vi "Point Style Read.vi"(4 "error in (no error)":errorcluster, 6 "Container State":T3, 7 "Display State In":T1) -> (0 "error out":errorcluster, 2 "Value":u8, 3 "Display State Out":T1)   [LabVIEW 2020, in "XY Plot Matrix.xctl"]
uses:
  <vilib>/Math Plots/2D Math Plots/XY Plot Matrix/XY Plot Matrix XCtrl/XY Plot Matrix.xctl
  <vilib>/_xctls/Container State.ctl
  <vilib>/Math Plots/2D Math Plots/XY Plot Matrix/XY Plot Matrix XCtrl/State.ctl
  <vilib>/Math Plots/2D Math Plots/XY Plot Matrix/XY Plot Matrix/XY Plot Matrix.lvclass
  e:/builds/penguin/labview/branches/2020/dev/dist/vi.lib/Math Plots/2D Math Plots/2D Plot/2D Plot/2D Plot.lvclass
  <vilib>/Math Plots/2D Math Plots/2D Plot/Action String/XYPlotMatrix Ctrl Act Queue.ctl
  <vilib>/Math Plots/2D Math Plots/2D Plot/Action String/XYPlotMatrix Ctrl Act Cluster.ctl
  <vilib>/Math Plots/2D Math Plots/2D Plot/Action String/2DMathPlot State Class.ctl
  <vilib>/Math Plots/2D Math Plots/2D Plot/2D Plot/2D Plot.lvclass
  <vilib>/_xctls/XControlSupport.lvlib
panel:
  # "Replace the Value Indicator below with an Indicator of desired type.\nDo not remove this Indicator or the others from the connector pane. \nDo not change the connector pane pattern.\nThe Value Indicator should always be the second terminal from top on the output side in the connector pane."
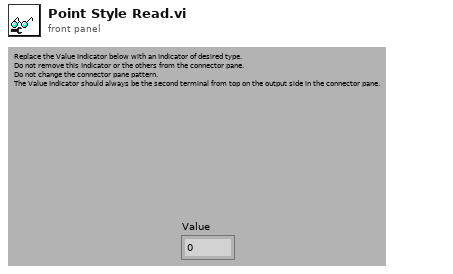
[diagram p1: front panel]
types:
  T1 = typedef "XY Plot Matrix.xctl/State.ctl" = cluster{"XY Plot Matrix.lvclass":refnum<class "XY Plot Matrix.lvclass">, "Control Ref Queue":T2, "Main Frame Color":u32}
  T2 = typedef "XYPlotMatrix Ctrl Act Queue.ctl" = refnum<queue>
  T3 = typedef "XControlSupport.lvlib/Container State.ctl" = cluster{"Indicator?":bool, "Run Mode?":bool, " Refnum":refnum<vi>}
  T4 = typedef "XY Plot Matrix.lvclass/Plotmatrix Property Array Cluster.ctl" = cluster{"Plotmatrix Property Array":T5, "Active Position":T9}
  T5 = typedef "XY Plot Matrix.lvclass/Plotmatrix Property Array.ctl" = T6[][]
  T6 = typedef "XY Plot Matrix.lvclass/Plotmatrix Property.ctl" = cluster{"Plot Property Array":T7}
  T7 = typedef "2D Plot.lvclass/Plot Property Array.ctl" = T8[]
  T8 = typedef "2D Plot.lvclass/Plot Property.ctl" = cluster{"Bar Plot Style":u8, "DigitalLineStyle":u8, "TransitionLocation":u8, "Transition Type":u8, "Fill To":i16, "Fill/Pt. Color":u32, "Label Style":u8, "Line Style":u8, "Line Width":u8, "Plot Color":u32, "Plot Interpolation":u8, "Plot Name":string, "Point Style":u8, "Visible?":bool, "XScaleIdx":u32, "YScaleIdx":u32}
  T9 = typedef "XY Plot Matrix.lvclass/Active Position.ctl" = cluster{"Row":i32, "Column":i32}
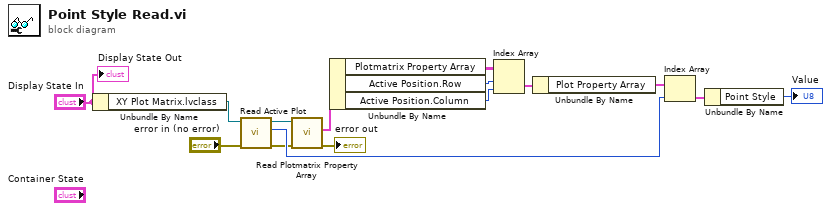
[diagram p0: block diagram]
diagram:
  n1 = Unbundle By Name("Display State In") -> ("XY Plot Matrix.lvclass"=w9:refnum<class "XY Plot Matrix.lvclass">)
  n2 = call <vilib>:"Read Active Plot.vi"("error in (no error)"="error in (no error)", "2D Plot.lvclass in"=w9) -> ("error out"=w5:errorcluster, "Active Plot"=w7:i32, "2D Plot.lvclass out"=w8:refnum<class "XY Plot Matrix.lvclass">)  [unwired: 7 out]
  n3 = call <vilib>:"Read Plotmatrix Property Array.vi"("error in (no error)"=w5, "2D Plotmatrix.lvclass in"=w8) -> ("error out"=→"error out":errorcluster, "Plotmatrix Property Array Cluster"=w15:T4)  [unwired: 8 out]
  n4 = Unbundle By Name(w15) -> ("Plotmatrix Property Array"=w14:T5, "Active Position.Row"=w13:i32, "Active Position.Column"=w12:i32)
  n5 = Index Array(array=w14, index (row)=w13, index (col)=w12) -> (element=w11:T6)
  n6 = Unbundle By Name(w11) -> ("Plot Property Array"=w10:T7)
  n7 = Index Array(array=w10, index=w7) -> (element=w6:T8)
  n8 = Unbundle By Name(w6) -> ("Point Style"=→"Value":u8)
  "Display State Out" <- "Display State In"
